vi "marble counter 2.vi"(0 "Trash Marble-in":dbl, 1 "White Large-in":dbl, 3 "White Small-in":dbl, 4 "Red Large-in":dbl, 5 "Red small-in":dbl, 7 "Blue Large-in":dbl, 8 "blue small-in":dbl, 9 "HDPE-in":dbl, 10 "Steel -in":dbl, 12 "Marble Type Input":dbl, 13 "No marble Detected-in":dbl) -> (14 "Trash Marble-out":dbl, 15 "No marble Detected-out":dbl, 16 "White Large-out":dbl, 17 "Steel-out":dbl, 20 "White small-out":dbl, 21 "Red Large-out":dbl, 23 "Red small-out":dbl, 24 "blue large-out":dbl, 25 "blue small-out":dbl, 27 "HDPE-out":dbl)   [LabVIEW 2016]
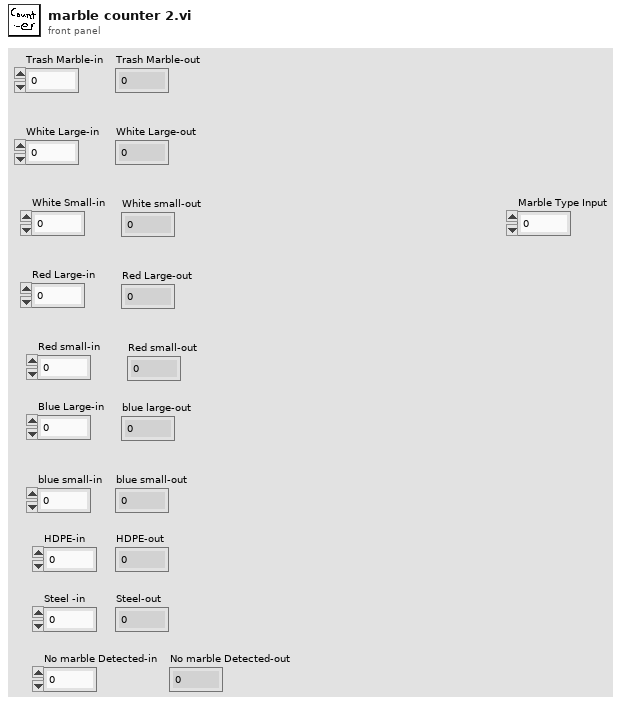
[diagram p1: front panel]
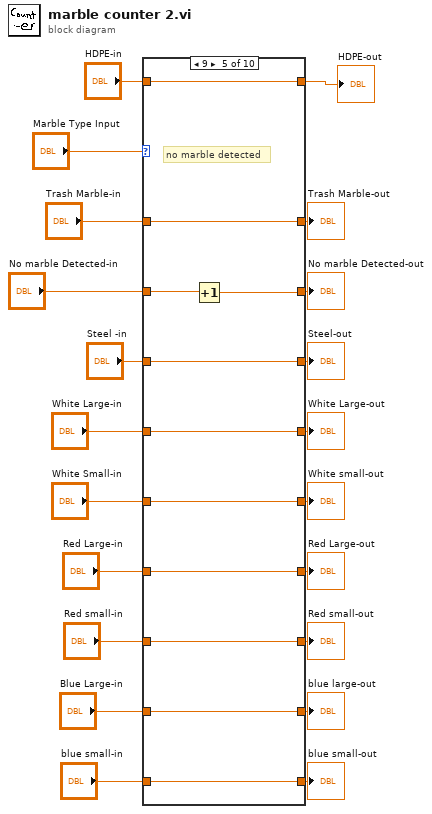
[diagram p0: block diagram]
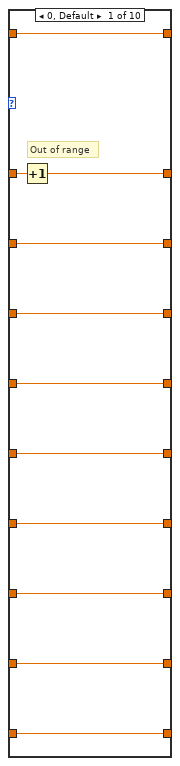
[diagram p2: hidden frame]
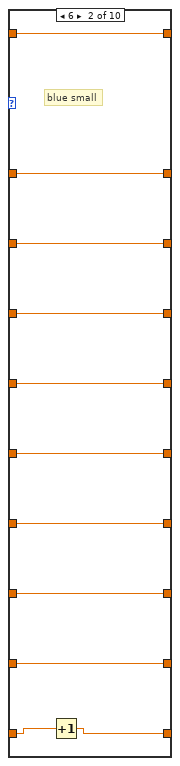
[diagram p3: hidden frame]
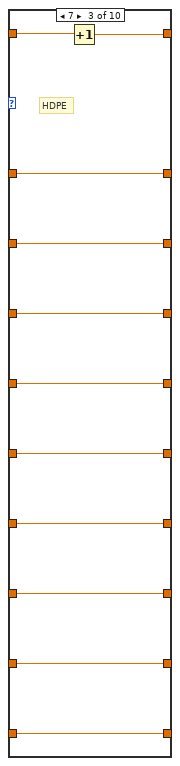
[diagram p4: hidden frame]
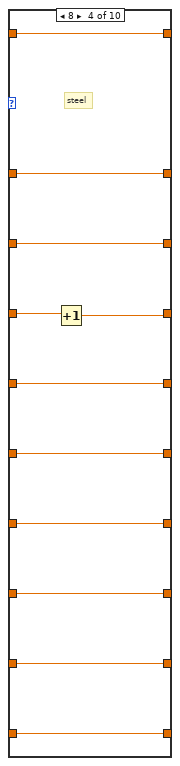
[diagram p5: hidden frame]
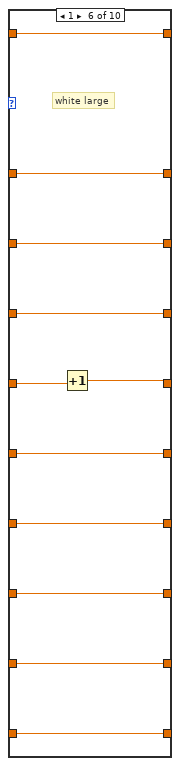
[diagram p6: hidden frame]
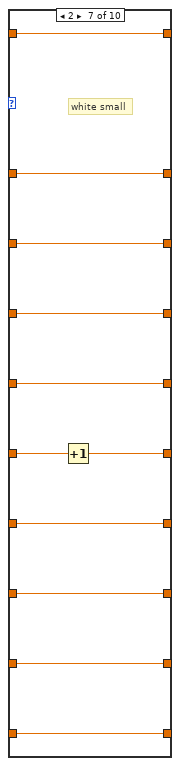
[diagram p7: hidden frame]
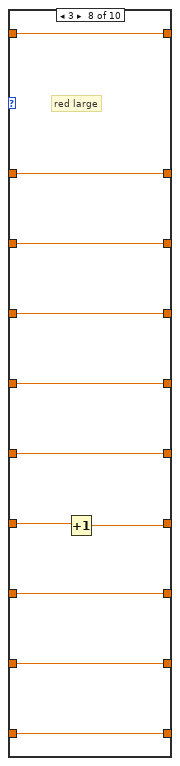
[diagram p8: hidden frame]
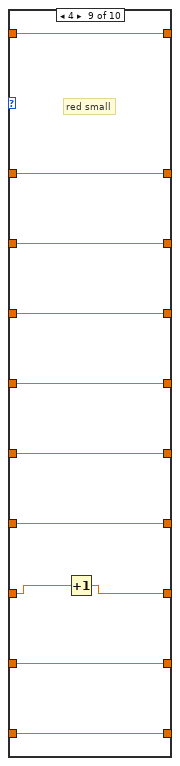
[diagram p9: hidden frame]
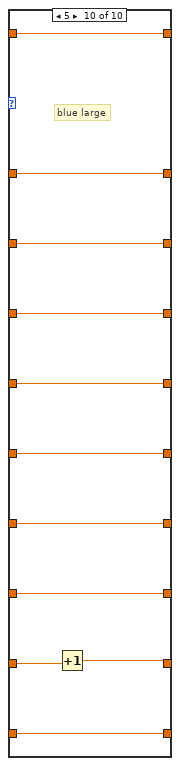
[diagram p10: hidden frame]
diagram:
  n1 = case shown="9" "Marble Type Input" {
    tunnel: "Trash Marble-in" -> [w32 w42 w52 w64 w75 w86 w97 w108 w119 w130]
    tunnel: [w31 w42 w52 w64 w75 w86 w97 w108 w119 w130] -> w9
    tunnel: [w30 w39 w49 w60 w71 w82 w94 w105 w116 w127] -> w6
    tunnel: "White Large-in" -> [w30 w39 w49 w60 w71 w83 w94 w105 w116 w127]
    tunnel: [w29 w38 w48 w59 w70 w81 w92 w104 w115 w126] -> w5
    tunnel: "White Small-in" -> [w29 w38 w48 w59 w70 w81 w93 w104 w115 w126]
    tunnel: [w28 w37 w47 w58 w69 w80 w91 w102 w114 w125] -> w4
    tunnel: "Red Large-in" -> [w28 w37 w47 w58 w69 w80 w91 w103 w114 w125]
    tunnel: "Red small-in" -> [w27 w36 w46 w57 w68 w79 w90 w101 w113 w124]
    tunnel: [w27 w36 w46 w57 w68 w79 w90 w101 w112 w124] -> w3
    tunnel: "Blue Large-in" -> [w26 w35 w45 w56 w67 w78 w89 w100 w111 w123]
    tunnel: [w26 w35 w45 w56 w67 w78 w89 w100 w111 w122] -> w2
    tunnel: "blue small-in" -> [w25 w34 w44 w55 w66 w77 w88 w99 w110 w121]
    tunnel: [w25 w33 w44 w55 w66 w77 w88 w99 w110 w121] -> w1
    tunnel: [w24 w43 w53 w65 w76 w87 w98 w109 w120 w131] -> w10
    tunnel: "HDPE-in" -> [w24 w43 w54 w65 w76 w87 w98 w109 w120 w131]
    tunnel: [w23 w40 w50 w61 w72 w84 w95 w106 w117 w128] -> w7
    tunnel: "Steel -in" -> [w23 w40 w50 w62 w72 w84 w95 w106 w117 w128]
    tunnel: [w22 w41 w51 w63 w73 w85 w96 w107 w118 w129] -> w8
    tunnel: "No marble Detected-in" -> [w22 w41 w51 w63 w74 w85 w96 w107 w118 w129]
    frame 0, Default {
      # "Out of range"
      n2 = Increment(x=w32) -> (x+1=w31:dbl)
    }
    frame 6 {
      # "blue small"
      n3 = Increment(x=w34) -> (x+1=w33:dbl)
    }
    frame 7 {
      # "HDPE"
      n4 = Increment(x=w54) -> (x+1=w53:dbl)
    }
    frame 8 {
      # "steel"
      n5 = Increment(x=w62) -> (x+1=w61:dbl)
    }
    frame 9 {
      # "no marble detected"
      n6 = Increment(x=w74) -> (x+1=w73:dbl)
    }
    frame 1 {
      # "white large"
      n7 = Increment(x=w83) -> (x+1=w82:dbl)
    }
    frame 2 {
      # "white small"
      n8 = Increment(x=w93) -> (x+1=w92:dbl)
    }
    frame 3 {
      # "red large"
      n9 = Increment(x=w103) -> (x+1=w102:dbl)
    }
    frame 4 {
      # "red small"
      n10 = Increment(x=w113) -> (x+1=w112:dbl)
    }
    frame 5 {
      # "blue large"
      n11 = Increment(x=w123) -> (x+1=w122:dbl)
    }
  }
  "HDPE-out" <- w10
  "Trash Marble-out" <- w9
  "No marble Detected-out" <- w8
  "Steel-out" <- w7
  "White Large-out" <- w6
  "White small-out" <- w5
  "Red Large-out" <- w4
  "Red small-out" <- w3
  "blue large-out" <- w2
  "blue small-out" <- w1
